vi "STS-Used_09_11_12a_JW.vi"(10 "Id Used":dbl[](array[numeric]), 11 "Vg-Used":dbl[](array[numeric])) -> (3 "STS":dbl)   [LabVIEW 2011]
uses:
  <vilib>/Analysis/NI_AALPro.lvlib
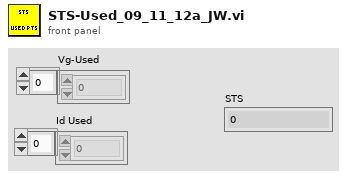
[diagram p1: front panel]
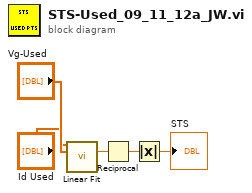
[diagram p0: block diagram]
diagram:
  n1 = call <vilib>:"Linear Fit.vi"("Y"="Id Used", "X"="Vg-Used") -> ("slope"=w5:dbl)  [unwired: 9 in, 4 out]
  n2 = Reciprocal(x=w5) -> (1/x=w4:dbl)
  n3 = Absolute Value(x=w4) -> (abs(x)=→"STS":dbl)
